vi "SetGetCoordSystemType - Test.vi"() -> ()   [LabVIEW 2017]
uses:
  AT901 API/TypeDefinitions/ES_CoordinateSystemType.ctl
panel:
  out "ES_CoordinateSystemType 2":T1
  in  "ES_CoordinateSystemType":T1
  out "error out":errorcluster
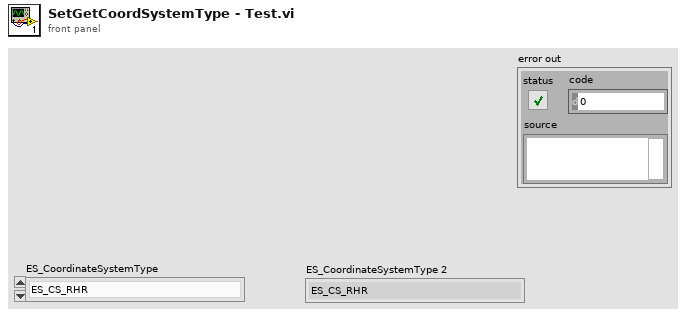
[diagram p1: front panel]
types:
  T1 = typedef "ES_CoordinateSystemType.ctl" = enum32{"ES_CS_RHR", "ES_CS_LHRX", "ES_CS_LHRY", "ES_CS_LHRZ", "ES_CS_CCW", "ES_CS_CCC", "ES_CS_SCW", "ES_CS_SCC"}
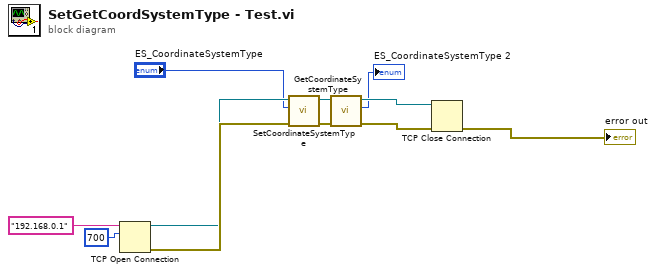
[diagram p0: block diagram]
diagram:
  n1 = TCP Open Connection(address="192.168.0.1", remote port or service name=u16 700) -> (connection ID=w3:refnum<k5>, error out=w6:errorcluster)  [unwired: 3 in]
  n2 = call "SetCoordinateSystemType.vi"("error in (no error)"=w6, "ES_CoordinateSystemType"="ES_CoordinateSystemType", "TCP Network Connection in"=w3) -> ("error out"=w7:errorcluster, "TCP Network Connection out"=w8:refnum<k5>)  [unwired: 5 in, 2 out]
  n3 = call "GetCoordinateSystemType.vi"("error in (no error)"=w7, "TCP Network Connection in"=w8) -> ("error out"=w5:errorcluster, "ES_CoordinateSystemType"=→"ES_CoordinateSystemType 2":T1, "TCP Network Connection out"=w4:refnum<k5>)  [unwired: 5 in, 2 out]
  n4 = TCP Close Connection(connection ID=w4, error in (no error)=w5) -> (error out=→"error out":errorcluster)  [unwired: 1 in, 1 out]
